vi "Control_Array_QMH_Init.vi"() -> (3 "Init setting":T1(array[cluster]))   [LabVIEW 2015]
uses:
  Control_IOControl.ctl
  Control_CameraControl.ctl
  Control_ImageControl.ctl
  Control_Inspection.ctl
  Control_FileControl.ctl
  Control_MachineVerification.ctl
  Control_LightControl.ctl
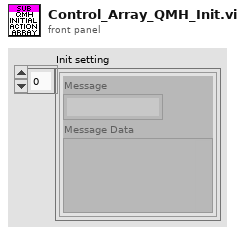
[diagram p1: front panel]
types:
  T1 = cluster{"Message":string, "Message Data":variant}[]
  T2 = typedef "Control_LightControl.ctl" = enum16{"1.光源控制-初始化", "2.光源控制-光源開啟", "3.光源控制-光源關閉", "4.光源控制-通訊關閉"}
  T3 = cluster{"Message":string, "Message Data":variant}
  T4 = typedef "Control_FileControl.ctl" = enum16{"1.檔案-初始化", "2.檔案-儲存檔案", "3.檔案-開啟檔案", "4.檔案-匯入檔案"}
  T5 = typedef "Control_MachineVerification.ctl" = enum16{"1.機台驗證-初始化", "2.機台驗證-檢測"}
  T6 = typedef "Control_Inspection.ctl" = enum16{"1.檢測-初始化", "2.浪代-浪代"}
  T7 = typedef "Control_ImageControl.ctl" = enum16{"1.影像-初始化", "2.影像-更新影像", "3.影像-儲存影像"}
  T8 = typedef "Control_CameraControl.ctl" = enum16{"1.相機-初始化", "2.相機-取像", "3.相機-關閉"}
  T9 = typedef "Control_IOControl.ctl" = enum16{"1.IO-初始化", "2. Set Point(EOT On)", "3.Set Point(EOT Off)", "4.Get Point(SOT)"}
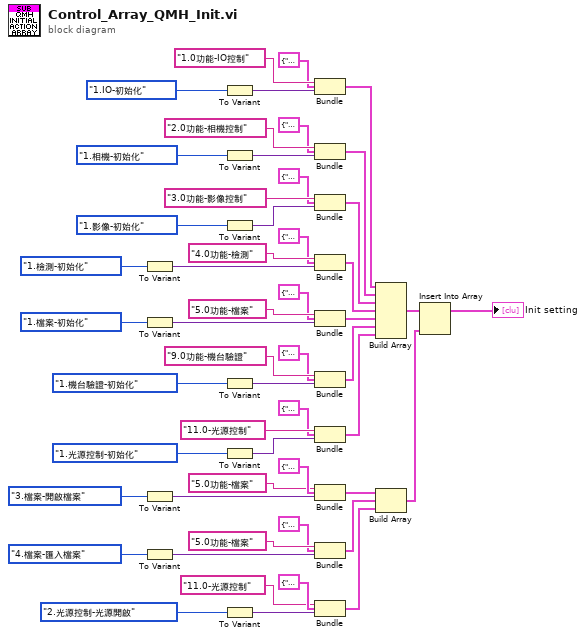
[diagram p0: block diagram]
diagram:
  n1 = To Variant(anything=Control_Inspection."1.檢測-初始化" ("4.0功能-檢測")) -> (Variant=w25:variant)
  n2 = To Variant(anything=Control_FileControl."1.檔案-初始化" ("5.0功能-檔案")) -> (Variant=w26:variant)
  n3 = To Variant(anything=Control_FileControl."3.檔案-開啟檔案" ("5.0功能-檔案")) -> (Variant=w39:variant)
  n4 = To Variant(anything=Control_FileControl."4.檔案-匯入檔案" ("5.0功能-檔案")) -> (Variant=w40:variant)
  n5 = To Variant(anything=Control_IOControl."1.IO-初始化" ("1.0 功能-IO控制")) -> (Variant=w22:variant)
  n6 = To Variant(anything=Control_CameraControl."1.相機-初始化" ("2.0功能-相機控制")) -> (Variant=w23:variant)
  n7 = To Variant(anything=Control_ImageControl."1.影像-初始化" ("3.0功能-影像控制")) -> (Variant=w24:variant)
  n8 = To Variant(anything=Control_MachineVerification."1.機台驗證-初始化" ("9.0功能-機台驗證")) -> (Variant=w27:variant)
  n9 = To Variant(anything=Control_LightControl."1.光源控制-初始化" ("11.0-光源控制")) -> (Variant=w28:variant)
  n10 = To Variant(anything=Control_LightControl."2.光源控制-光源開啟" ("11.0-光源控制")) -> (Variant=w44:variant)
  n11 = Bundle(cluster=T3 {"Message"="", "Message Data"=variant} ("element"), "Message"="1.0功能-IO控制" ("Label.Text"), "Message Data"=w22) -> (w29:T3)
  n12 = Bundle(cluster=T3 {"Message"="", "Message Data"=variant} ("element"), "Message"="2.0功能-相機控制" ("Label.Text"), "Message Data"=w23) -> (w30:T3)
  n13 = Bundle(cluster=T3 {"Message"="", "Message Data"=variant} ("element"), "Message"="3.0功能-影像控制" ("Label.Text"), "Message Data"=w24) -> (w31:T3)
  n14 = Bundle(cluster=T3 {"Message"="", "Message Data"=variant} ("element"), "Message"="4.0功能-檢測" ("Label.Text"), "Message Data"=w25) -> (w32:T3)
  n15 = Bundle(cluster=T3 {"Message"="", "Message Data"=variant} ("element"), "Message"="5.0功能-檔案" ("Label.Text"), "Message Data"=w26) -> (w33:T3)
  n16 = Bundle(cluster=T3 {"Message"="", "Message Data"=variant} ("element"), "Message"="9.0功能-機台驗證" ("Label.Text"), "Message Data"=w27) -> (w34:T3)
  n17 = Bundle(cluster=T3 {"Message"="", "Message Data"=variant} ("element"), "Message"="11.0-光源控制" ("Label.Text"), "Message Data"=w28) -> (w35:T3)
  n18 = Bundle(cluster=T3 {"Message"="", "Message Data"=variant} ("element"), "Message"="5.0功能-檔案" ("Label.Text"), "Message Data"=w39) -> (w48:T3)
  n19 = Bundle(cluster=T3 {"Message"="", "Message Data"=variant} ("element"), "Message"="5.0功能-檔案" ("Label.Text"), "Message Data"=w40) -> (w49:T3)
  n20 = Bundle(cluster=T3 {"Message"="", "Message Data"=variant} ("element"), "Message"="11.0-光源控制" ("Label.Text"), "Message Data"=w44) -> (w50:T3)
  n21 = Build Array(w29, w30, w31, w32, w33, w34, w35) -> (w51:T1)
  n22 = Build Array(w48, w49, w50) -> (w52:T1)
  n23 = Insert Into Array(array=w51, new element=w52) -> (→"Init setting":T1)  [unwired: 1 in]
